vi "FFT特征.vi"(6 "低频点":i32, 7 "高频点":i32, 8 "样板2":dbl[](graph), 9 "样板":dbl[](graph), 10 "幅度误差":dbl, 11 "输入":dbl[](graph)) -> (1 "主频":i32, 2 "样板2匹配":bool[](array[boolean]), 3 "样板1匹配":bool[](array[boolean]))   [LabVIEW 2014]
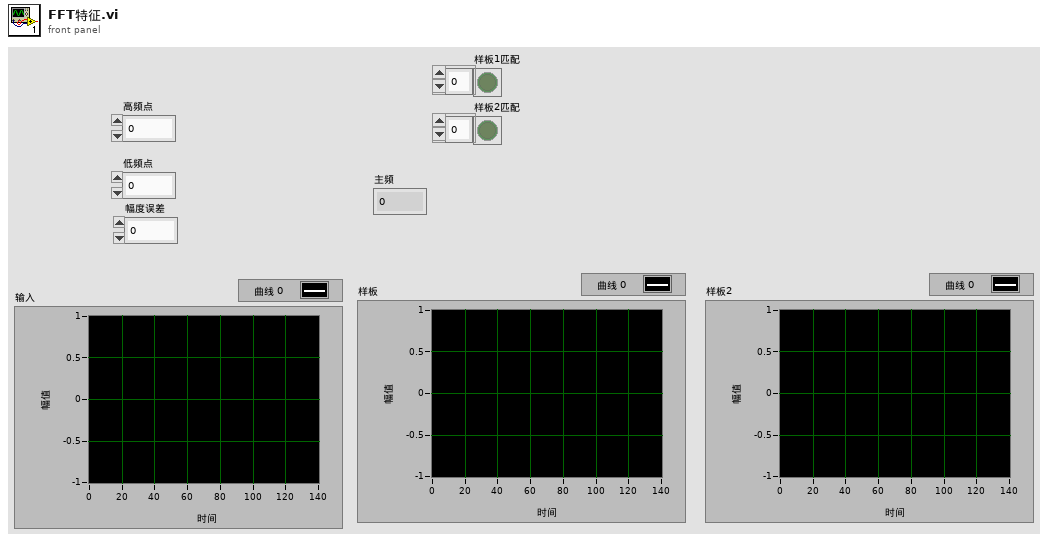
[diagram p1: front panel]
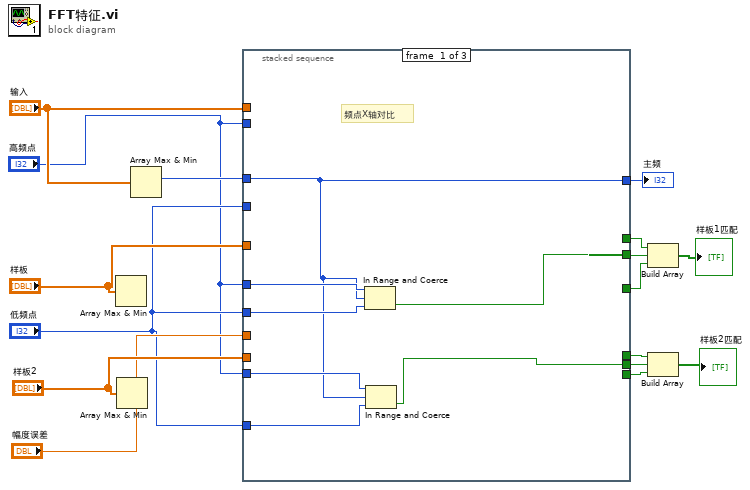
[diagram p0: block diagram]
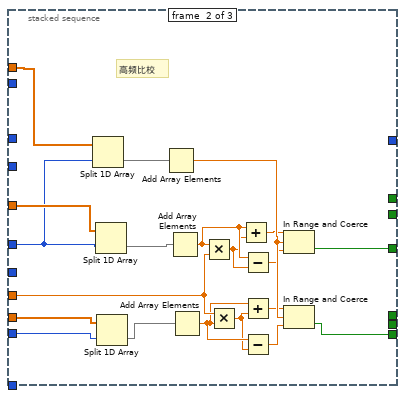
[diagram p2: hidden frame]
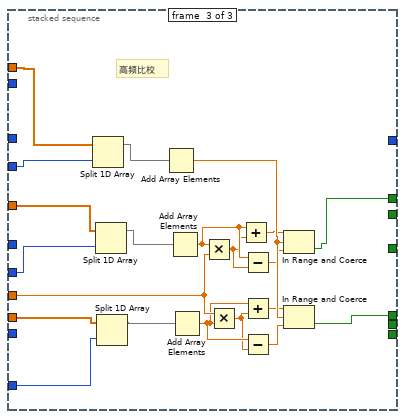
[diagram p3: hidden frame]
diagram:
  n1 = Array Max & Min(array="样板") -> ()  [unwired: 4 out]
  n2 = Array Max & Min(array="样板2") -> ()  [unwired: 4 out]
  n3 = Array Max & Min(array="输入") -> (max index (indices)=w14:i32)  [unwired: 3 out]
  n4 = stacked-sequence {
    tunnel: "高频点" -> [w23 w39 _]
    tunnel: "低频点" -> [w22 _ w46]
    tunnel: "高频点" -> [w21 w40 _]
    tunnel: "低频点" -> [w20 _ w45]
    tunnel: w14 -> [w17 _ _]
    tunnel: "样板" -> [_ w41 w62]
    tunnel: "样板2" -> [_ w42 w63]
    tunnel: "高频点" -> [_ _ _]
    tunnel: "低频点" -> [_ _ w44]
    tunnel: "输入" -> [_ w43 w64]
    tunnel: "幅度误差" -> [_ w30 w56]
    tunnel: [w19 _ _] -> w11
    tunnel: [w18 _ _] -> w10
    tunnel: [_ w25 _] -> w5
    tunnel: [_ w24 _] -> w4
    tunnel: [_ _ w51] -> w3
    tunnel: [_ _ w50] -> w2
    tunnel: [w17 _ _] -> w1
    frame #0 {
      # "频点X轴对比"
      n5 = In Range and Coerce(upper limit=w21, x=w17, lower limit=w20) -> (In Range?=w19:bool)  [unwired: 1 out]
      n6 = In Range and Coerce(upper limit=w23, x=w17, lower limit=w22) -> (In Range?=w18:bool)  [unwired: 1 out]
    }
    frame #1 {
      # "高频比校"
      n7 = Split 1D Array(array=w43, index=w40) -> (second subarray=w37:dbl[])  [unwired: 1 out]
      n8 = Split 1D Array(array=w41, index=w40) -> (second subarray=w38:dbl[])  [unwired: 1 out]
      n9 = Split 1D Array(array=w42, index=w39) -> (second subarray=w36:dbl[])  [unwired: 1 out]
      n10 = Add Array Elements(numeric array=w37) -> (sum=w35:dbl)
      n11 = Add Array Elements(numeric array=w38) -> (sum=w33:dbl)
      n12 = Add Array Elements(numeric array=w36) -> (sum=w27:dbl)
      n13 = Multiply(x=w33, y=w30) -> (x*y=w32:dbl)
      n14 = Multiply(x=w30, y=w27) -> (x*y=w26:dbl)
      n15 = Add(x=w33, y=w32) -> (x+y=w34:dbl)
      n16 = Subtract(x=w33, y=w32) -> (x-y=w31:dbl)
      n17 = Add(x=w27, y=w26) -> (x+y=w29:dbl)
      n18 = Subtract(x=w27, y=w26) -> (x-y=w28:dbl)
      n19 = In Range and Coerce(upper limit=w34, x=w35, lower limit=w31) -> (In Range?=w24:bool)  [unwired: 1 out]
      n20 = In Range and Coerce(upper limit=w29, x=w35, lower limit=w28) -> (In Range?=w25:bool)  [unwired: 1 out]
    }
    frame #2 {
      # "高频比校"
      n21 = Split 1D Array(array=w64, index=w44) -> (first subarray=w47:dbl[])  [unwired: 1 out]
      n22 = Split 1D Array(array=w62, index=w45) -> (first subarray=w48:dbl[])  [unwired: 1 out]
      n23 = Split 1D Array(array=w63, index=w46) -> (first subarray=w49:dbl[])  [unwired: 1 out]
      n24 = Add Array Elements(numeric array=w47) -> (sum=w61:dbl)
      n25 = Add Array Elements(numeric array=w48) -> (sum=w59:dbl)
      n26 = Add Array Elements(numeric array=w49) -> (sum=w53:dbl)
      n27 = Multiply(x=w59, y=w56) -> (x*y=w58:dbl)
      n28 = Multiply(x=w56, y=w53) -> (x*y=w52:dbl)
      n29 = Add(x=w59, y=w58) -> (x+y=w60:dbl)
      n30 = Subtract(x=w59, y=w58) -> (x-y=w57:dbl)
      n31 = Add(x=w53, y=w52) -> (x+y=w55:dbl)
      n32 = Subtract(x=w53, y=w52) -> (x-y=w54:dbl)
      n33 = In Range and Coerce(upper limit=w60, x=w61, lower limit=w57) -> (In Range?=w51:bool)  [unwired: 1 out]
      n34 = In Range and Coerce(upper limit=w55, x=w61, lower limit=w54) -> (In Range?=w50:bool)  [unwired: 1 out]
    }
  }
  "主频" <- w1
  n35 = Build Array(w3, w11, w4) -> (→"样板1匹配":bool[])
  n36 = Build Array(w2, w10, w5) -> (→"样板2匹配":bool[])
